vi "Sys Exec Error Wrapper.vi"(7 "command line":string, 8 "error in (no error)":errorcluster, 10 "standard error":string, 11 "standard output":string) -> (0 "error out":errorcluster)   [LabVIEW 2021, in "CIFCoreCommon.lvlib"]
uses:
  CIFCoreCommon.lvlib
  Typedef/Errors.ctl
  Add Error Core.vi
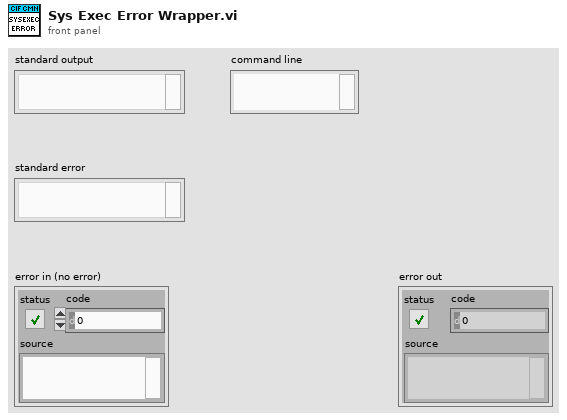
[diagram p1: front panel]
types:
  T1 = typedef "CIFCoreCommon.lvlib/Errors.ctl" = enum16{"Invalid Clock ID", "Long Sleep", "gRPC Server Not Found", "Config Parse", "Timestamp Wrap", "Delayed Execution", "Duplicate Channel", "Missing Channel", "Incorrect Type", "Flatten Error", "Unflatten Data", "Unique Name", "Plugin Not Found", "Plugin Type Not Found", "Plugin Version Not Found", "Manager Not Found", "Numerical Issue", "Time Jump", "Clock ID Match", "Channel Length", "Plugin Connection", "gRPC Server Connection", "PPL Name Match", "Build", "Config Log Parse", "Plugin Load", "UI Subpanel Load", "Python Name", "Invalid Name", "Unable to Change Ch Buffer", "Failed Kill", "Failed SysExec", "Function Not Implemented", "Load Timeout", "Invalid FTE", "Manager Crash"}
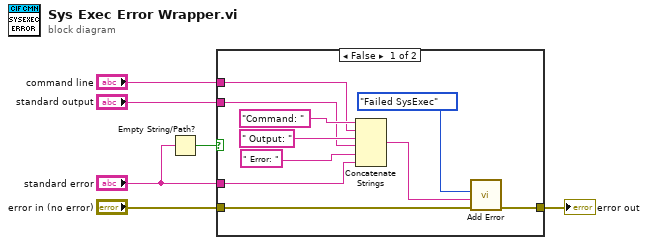
[diagram p0: block diagram]
diagram:
  n1 = Empty String/Path?(string/path="standard error") -> (empty?=w6:bool)
  n2 = case shown="False" w6 {
    tunnel: "error in (no error)" -> [w16 w17]
    tunnel: [w15 w17] -> w4
    tunnel: "standard error" -> [w11 _]
    tunnel: "command line" -> [w10 _]
    tunnel: "standard output" -> [w9 _]
    frame False {
      n3 = Concatenate Strings("Command: " ("string"), w10, " Output: " ("string"), w9, " Error: " ("string"), w11) -> (w8:string)
      n4 = call "Add Error.vi"("error in (no error)"=w16, "String to Append"=w8, "Error"=Errors."Failed SysExec") -> ("error out"=w15:errorcluster)  [unwired: 8 in]
    }
    frame True {
    }
  }
  "error out" <- w4
